vi "event_setup_pause.vi"(7 "NewVal":bool, 8 "error in":errorcluster, 9 "reference cluster in":T1, 11 "Boolean in":refnum<vi>) -> (0 "error out":errorcluster)   [LabVIEW 2016]
uses:
  Type Definitions/reference_cluster.ctl
  Type Definitions/vars_settings.ctl
  Type Definitions/stim_type.ctl
  Type Definitions/backlight_type.ctl
  Type Definitions/vars_runtime.ctl
  Type Definitions/data.ctl
  Type Definitions/notifier_elements_GUI.ctl
  Type Definitions/notifier_elements_DAQ.ctl
  Type Definitions/notifier_elements_write.ctl
  Type Definitions/control_references.ctl
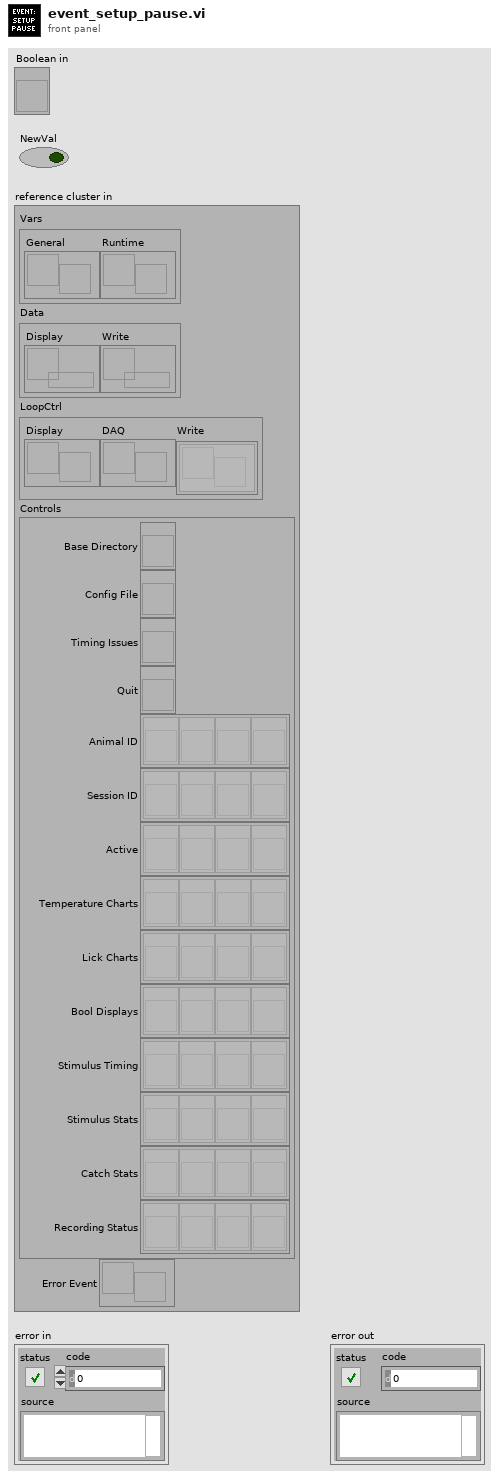
[diagram p1: front panel]
types:
  T1 = typedef "reference_cluster.ctl" = cluster{"Vars":cluster{"General":refnum<notifier>, "Runtime":refnum<notifier>}, "Data":cluster{"Display":refnum<queue>, "Write":refnum<queue>}, "LoopCtrl":cluster{"Display":refnum<notifier>, "DAQ":refnum<notifier>, "Write":refnum<notifier>[]}, "Controls":T2, "Error Event":refnum<user-event>}
  T2 = typedef "control_references.ctl" = cluster{"Base Directory":refnum<vi>, "Config File":refnum<vi>, "Timing Issues":refnum<vi>, "Quit":refnum<vi>, "Animal ID":refnum<vi>[], "Session ID":refnum<vi>[], "Active":refnum<vi>[], "Temperature Charts":refnum<vi>[], "Lick Charts":refnum<vi>[], "Bool Displays":refnum<vi>[], "Stimulus Timing":refnum<vi>[], "Stimulus Stats":refnum<vi>[], "Catch Stats":refnum<vi>[], "Recording Status":refnum<vi>[]}
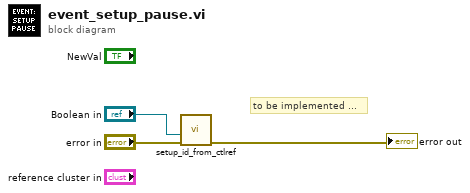
[diagram p0: block diagram]
diagram:
  # "to be implemented ..."
  n1 = call "setup_id_from_ctlref.vi"("error in"="error in", "Ctl Refnum"="Boolean in") -> ("error out"=→"error out":errorcluster)  [unwired: 6 in, 1 out]
